vi "Build_TDMS_File_Name.vi"(11 "Board_ID":string) -> ()   [LabVIEW 2017]
uses:
  Board_Global_Var.vi
  Measurement_Param_Global_Var.vi
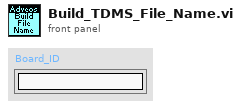
[diagram p1: front panel]
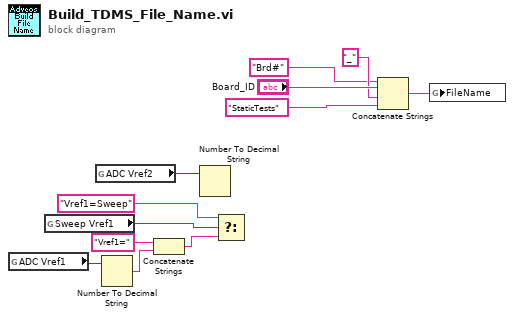
[diagram p0: block diagram]
diagram:
  n1 = global read "Measurement_Param_Global_Var.vi" "ADC Vref1"() -> (w12:u16)
  n2 = global read "Measurement_Param_Global_Var.vi" "Sweep Vref1"() -> (w4:bool)
  n3 = global read "Measurement_Param_Global_Var.vi" "ADC Vref2"() -> (w3:u16)
  n4 = Number To Decimal String(number=w12) -> (decimal integer string=w9:string)  [unwired: 1 in]
  n5 = Concatenate Strings("Vref1=" ("string"), w9) -> (w8:string)
  n6 = Number To Decimal String(number=w3) -> ()  [unwired: 1 in, 1 out]
  n7 = Select(t="Vref1=Sweep" ("string"), s=w4, f=w8) -> ()  [unwired: 1 out]
  n8 = Concatenate Strings("Brd#" ("File Name"), "Board_ID", "_" ("string"), "StaticTests" ("string")) -> (w11:string)
  n9 = global write "Board_Global_Var.vi" "FileName"(w11) -> ()
